vi "CNR project gradient and hessian.vi"(5 "bounds":T2, 7 "projected parameters":dbl[](array[numeric]), 8 "error in":errorcluster, 9 "Jacobian":T1, 10 "gradient":dbl[](array[numeric]), 11 "Hessian":T1) -> (0 "error out":errorcluster, 1 "projected jacobian":T1, 2 "projected gradient":dbl[](array[numeric]), 3 "projected Hessian":T1)   [LabVIEW 2020, in "NI_Gmath.lvlib"]
uses:
  <vilib>/gmath/NI_Gmath.lvlib
  <vilib>/Analysis/Matrix/Datatypes/RealMatrix.ctl
  <vilib>/Analysis/7linalg.llb/Create Special Real Matrix.vi
  <vilib>/Analysis/Matrix/Numeric/Add/Add - RM,RM.vi
  <vilib>/Analysis/NI_AALPro.lvlib
  <vilib>/Analysis/Matrix/NI_Matrix.lvlib
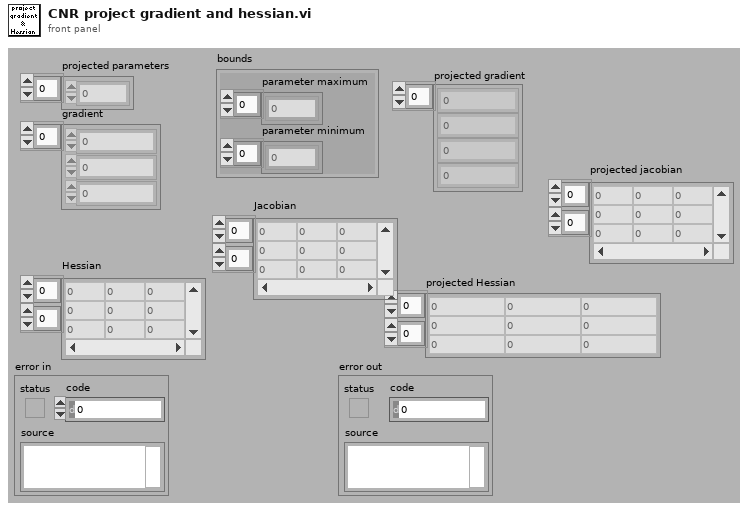
[diagram p1: front panel]
types:
  T1 = typedef "NI_Matrix.lvlib/RealMatrix.ctl" = dbl[][]
  T2 = cluster{"parameter minimum":dbl[], "parameter maximum":dbl[]}
  T3 = enum32{"Identity", "Diagonal", "Toepliz", "Vandermonde", "Companion"}
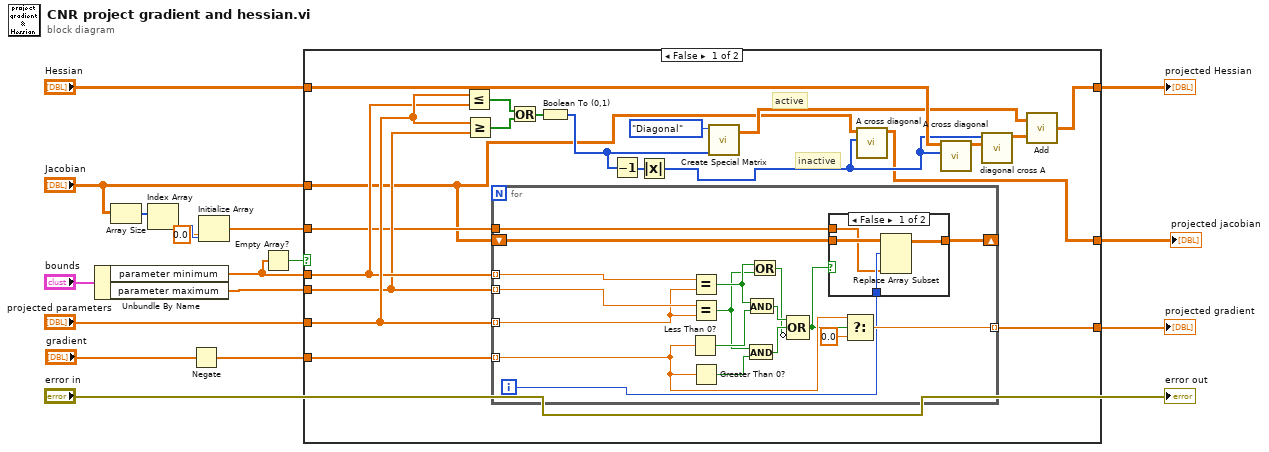
[diagram p0: block diagram]
diagram:
  n1 = Unbundle By Name("bounds") -> ("parameter minimum"=w10:dbl[], "parameter maximum"=w9:dbl[])
  n2 = Array Size(array="Jacobian") -> (size(s)=w5:i32[])
  n3 = Index Array(array=w5) -> (element=w4:i32)  [unwired: 1 in]
  n4 = Negate(x="gradient") -> (-x=w7:dbl[])
  n5 = Initialize Array(0.0 ("element"), w4) -> (w2:dbl[])
  n6 = Empty Array?(array=w10) -> (empty?=w8:bool)
  n7 = case shown="False" w8 {
    tunnel: "Hessian" -> [w36 w63]
    tunnel: [w32 w63] -> w16
    tunnel: w7 -> [w22 w62]
    tunnel: [w31 w62] -> w17
    tunnel: "projected parameters" -> [w26 _]
    tunnel: w10 -> [w25 _]
    tunnel: w9 -> [w24 _]
    tunnel: "Jacobian" -> [w19 w61]
    tunnel: w2 -> [w21 _]
    tunnel: [w18 w61] -> w1
    frame False {
      # "inactive"
      # "active"
      n8 = Less Or Equal?(x=w26, y=w25) -> (x <= y?=w29:bool[])
      n9 = Greater Or Equal?(x=w26, y=w24) -> (x >= y?=w28:bool[])
      n10 = for {
        tunnel: w22 -> [w48] mode=indexing
        tunnel: w25 -> [w53] mode=indexing
        tunnel: w24 -> [w55] mode=indexing
        tunnel: w26 -> [w54] mode=indexing
        tunnel: [w47] -> w31 mode=indexing
        shift-right: [w40] -> _
        shift-left: w19 -> [w41]
        tunnel: w21 -> [w39]
        i -> [w38]
        n11 = Less Than 0?(x=w48) -> (x < 0?=w52:bool)
        n12 = Equal?(x=w53, y=w54) -> (x = y?=w45:bool)
        n13 = Equal?(x=w55, y=w54) -> (x = y?=w44:bool)
        n14 = Greater Than 0?(x=w48) -> (x > 0?=w51:bool)
        n15 = And(x=w44, y=w51) -> (x .and. y?=w50:bool)
        n16 = And(x=w45, y=w52) -> (x .and. y?=w49:bool)
        n17 = Or(x=w45, y=w44) -> (x .or. y?=w43:bool)
        n18 = Compound Arithmetic op=OR(w49, w50, invert w43) -> (w42:bool)
        n19 = case shown="False" w42 {
          tunnel: w41 -> [w59 w60]
          tunnel: [w58 w60] -> w40
          tunnel: w39 -> [w56 _]
          tunnel: w38 -> [w57 _]
          frame False {
            n20 = Replace Array Subset(array=w59, new element=w56, index (row)=w57) -> (w58:T1)  [unwired: 1 in]
          }
          frame True {
          }
        }
        n21 = Select(t=w48, s=w42, f=0.0) -> (s? t:f=w47:dbl)
      }
      n22 = Or(x=w29, y=w28) -> (x .or. y?=w27:bool[])
      n23 = Boolean To (0,1)(Boolean=w27) -> (0, 1=w23:i16[])
      n24 = Decrement(x=w23) -> (x-1=w30:i16[])
      n25 = Absolute Value(x=w30) -> (abs(x)=w20:i16[])
      n26 = call-poly <vilib>:"Create Special Matrix.vi"("matrix type"=T3."Diagonal", "Input Vector1"=w23) -> ("Special Matrix"=w33:T1)  [unwired: 3 in, 1 out]
      n27 = call <vilib>:"A cross diagonal.vi"("diagonal"=w20, "A"=w19) -> ("Axdiagonal"=w18:T1)  [unwired: 9 in]
      n28 = call <vilib>:"A cross diagonal.vi"("diagonal"=w20, "A"=w36) -> ("Axdiagonal"=w35:T1)  [unwired: 9 in]
      n29 = call <vilib>:"diagonal cross A.vi"("A"=w35, "diagonal"=w20) -> ("diagonalxA"=w34:T1)  [unwired: 9 in]
      n30 = call-poly <vilib>:"Add.vi"("Real Matrix B"=w34, "Real Matrix A"=w33) -> ("A + B"=w32:T1)
    }
    frame True {
    }
  }
  "projected gradient" <- w17
  "projected Hessian" <- w16
  "projected jacobian" <- w1
  "error out" <- "error in"
